vi "MGI Bezier Inverse Time.vi"(1 "u":sgl format="%.2f", 2 "First k":i32, 3 "Bezier Control Points[]":sgl[](array[numeric]) format="%.4f") -> (0 "t":sgl format="%.2f")   [LabVIEW 2016]
doc: "Calculate a time from a block index and a 0..1 parameter. Actually performs an inverse Bezier function rather than a forward one, so u is first mapped linearly to the time range, then an inverse Bezier is calculated, and then the result is remapped into the time range.\n\nAuthored by David A. Moore\nsupport@mooregoodideas.com\nwww.mooregoodideas.com\n\nCopyright (c) 2010, Moore Good Ideas, Inc.\n\nAll rights reserved.\n\nRedistribution and use in source and binary forms, with or without modification, are permitted provided that the following conditions are met:\n\n * Redistributions of source code must retain the above copyright notice, this list of conditions and the following disclaimer.\n * Redistributions in binary form must reproduce the above copyright notice, this list of conditions and the following disclaimer in the documentation and/or other materials provided with the distribution.\n * Neither the name of Moore Good Ideas, Inc. nor the names of its contributors may be used to endorse or promote products derived from this software without specific prior written permission.\n\nTHIS SOFTWARE IS PROVIDED BY THE COPYRIGHT HOLDERS AND CONTRIBUTORS \"AS IS\" AND ANY EXPRESS OR IMPLIED WARRANTIES, INCLUDING, BUT NOT LIMITED TO, THE IMPLIED WARRANTIES OF MERCHANTABILITY AND FITNESS FOR A PARTICULAR PURPOSE ARE DISCLAIMED. IN NO EVENT SHALL THE COPYRIGHT OWNER OR CONTRIBUTORS BE LIABLE FOR ANY DIRECT, INDIRECT, INCIDENTAL, SPECIAL, EXEMPLARY, OR CONSEQUENTIAL DAMAGES (INCLUDING, BUT NOT LIMITED TO, PROCUREMENT OF SUBSTITUTE GOODS OR SERVICES; LOSS OF USE, DATA, OR PROFITS; OR BUSINESS INTERRUPTION) HOWEVER CAUSED AND ON ANY THEORY OF LIABILITY, WHETHER IN CONTRACT, STRICT LIABILITY, OR TORT (INCLUDING NEGLIGENCE OR OTHERWISE) ARISING IN ANY WAY OUT OF THE USE OF THIS SOFTWARE, EVEN IF ADVISED OF THE POSSIBILITY OF SUCH DAMAGE.i"
panel:
  # "k"
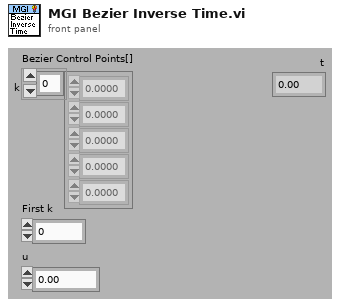
[diagram p1: front panel]
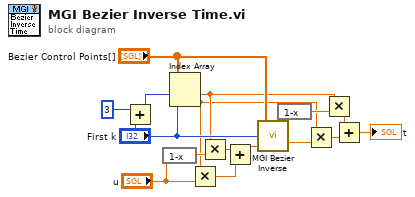
[diagram p0: block diagram]
diagram:
  n1 = Add(x=3, y="First k") -> (x+y=w15:i32)
  n2 = expression code="1-x"("u") -> (w13:sgl)
  n3 = Index Array(array="Bezier Control Points[]", index #1=w15, index #2="First k") -> (element #1=w7:sgl, element #2=w4:sgl)
  n4 = Multiply(x=w4, y="u") -> (x*y=w11:sgl)
  n5 = Multiply(x=w7, y=w13) -> (x*y=w12:sgl)
  n6 = Add(x=w12, y=w11) -> (x+y=w8:sgl)
  n7 = call <userlib>:"MGI Bezier Inverse.vi"("y"=w8, "First k"="First k", "Bezier Control Points[]"="Bezier Control Points[]") -> ("u"=w5:sgl)
  n8 = expression code="1-x"(w5) -> (w6:sgl)
  n9 = Multiply(x=w4, y=w5) -> (x*y=w3:sgl)
  n10 = Multiply(x=w7, y=w6) -> (x*y=w2:sgl)
  n11 = Add(x=w2, y=w3) -> (x+y=→"t":sgl)
